vi "REV2_Save_Config.vi"(7 "ID":u8, 8 "error in (no error)":errorcluster, 11 "VISA Refnum in":refnum<visa-resource-name>) -> (0 "error out":errorcluster, 3 "VISA Refnum out":refnum<visa-resource-name>)   [LabVIEW 2016, in "REV_2.lvlib"]
uses:
  REV_2.lvlib
  REV2_Instructions.ctl
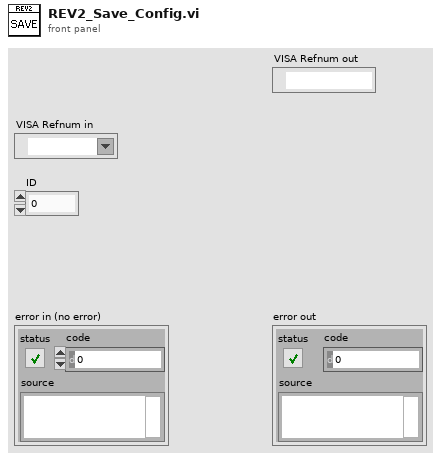
[diagram p1: front panel]
types:
  T1 = typedef "REV_2.lvlib/REV2_Instructions.ctl" = u8
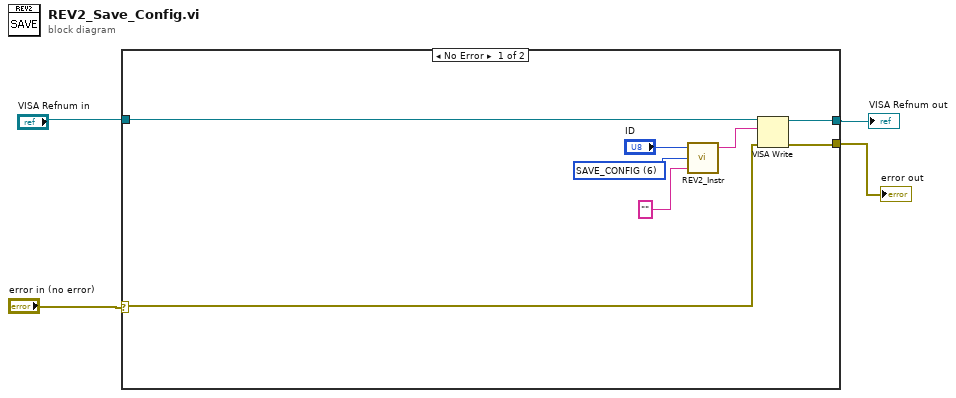
[diagram p0: block diagram]
diagram:
  n1 = case shown="No Error" "error in (no error)" {
    selector: "error in (no error)" -> [w6 w14]
    tunnel: [w11 w13] -> w4
    tunnel: [w10 w14] -> w3
    tunnel: "VISA Refnum in" -> [w7 w13]
    frame No Error {
      w12 = T1 6 items=["PING"=1, "READ_STAT"=2, "WRITE_STAT"=3, "READ_CONFIG"=4, "WRITE_CONFIG"=5, "SAVE_CONFIG"=6] ("Instruction")
      n2 = call "REV2_Instr.vi"("Parameter"="", "Instruction"=w12, "ID"="ID") -> ("Output"=w9:string)  [unwired: 2 in]
      n3 = VISA Write(VISA resource name=w7, write buffer=w9, error in (no error)=w6) -> (VISA resource name out=w11:refnum<visa-resource-name>, error out=w10:errorcluster)  [unwired: 1 out]
    }
    frame Error {
    }
  }
  "VISA Refnum out" <- w4
  "error out" <- w3
